vi "time elapsed.vi"(10 "%Completed":dbl=100.0 format="%#_13g", 11 "Start":dbl=3666.0 format="%#_13g") -> (0 "Minuites 2":dbl, 1 "Hours 2":dbl, 2 "Seconds":dbl, 3 "Minuites":dbl, 4 "Seconds 2":dbl, 5 "Hours":dbl)   [LabVIEW 2023, in "User Interface.lvlib"]
uses:
  User Interface.lvlib
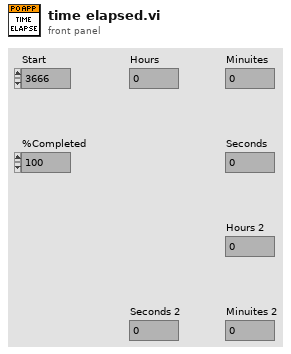
[diagram p1: front panel]
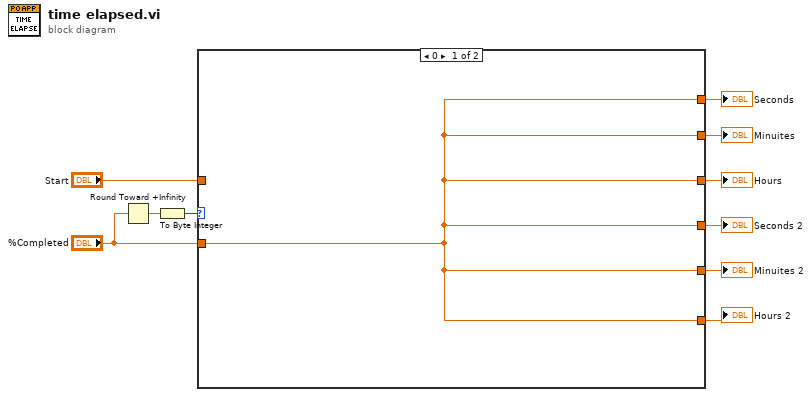
[diagram p0: block diagram]
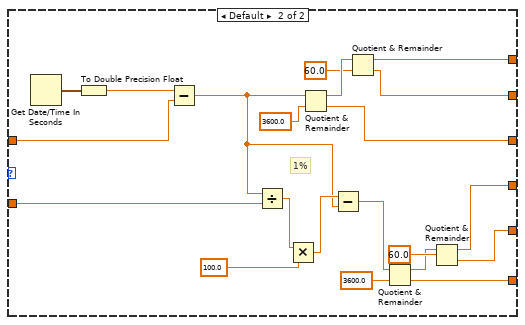
[diagram p2: hidden frame]
diagram:
  n1 = Round Toward +Infinity(x="%Completed") -> (ceil(x): smallest int >= x=w1:dbl)
  n2 = To Byte Integer(number=w1) -> (8bit integer=w4:i8)
  n3 = case shown="0" w4 {
    tunnel: [w11 w27] -> w10
    tunnel: [w11 w26] -> w9
    tunnel: [w11 w25] -> w8
    tunnel: [w11 w24] -> w7
    tunnel: [w11 w23] -> w6
    tunnel: [w11 w22] -> w5
    tunnel: "Start" -> [_ w12]
    tunnel: "%Completed" -> [w11 w17]
    frame 0 {
    }
    frame Default {
      # "1%"
      n4 = Get Date/Time In Seconds() -> (seconds since 1Jan1904=w32:timestamp)
      n5 = To Double Precision Float(number=w32) -> (double precision float=w31:dbl)
      n6 = Subtract(x=w31, y=w12) -> (x-y=w13:dbl)
      n7 = Divide(x=w13, y=w17) -> (x/y=w16:dbl)
      n8 = Multiply(x=w16, y=100.0) -> (x*y=w15:dbl)
      n9 = Quotient & Remainder(x=w13, y=3600.0) -> (x-y*floor(x/y)=w29:dbl, floor(x/y)=w27:dbl)
      n10 = Subtract(x=w15, y=w13) -> (x-y=w14:dbl)
      n11 = Quotient & Remainder(x=w29, y=60.0) -> (x-y*floor(x/y)=w25:dbl, floor(x/y)=w26:dbl)
      n12 = Quotient & Remainder(x=w14, y=3600.0) -> (x-y*floor(x/y)=w20:dbl, floor(x/y)=w22:dbl)
      n13 = Quotient & Remainder(x=w20, y=60.0) -> (x-y*floor(x/y)=w24:dbl, floor(x/y)=w23:dbl)
    }
  }
  "Hours" <- w10
  "Minuites" <- w9
  "Seconds" <- w8
  "Hours 2" <- w5
  "Minuites 2" <- w6
  "Seconds 2" <- w7
